vi "Window relative size to pixel size.vi"(8 "Border (px)":i16=4, 9 "Height (px)":i16=1920, 10 "Width (px)":i16=1920, 11 "Window Relative Size (%)":T2 {"Bottom (%)" format="%.2f"; "Top (%)" format="%.2f"; "Right (%)" format="%.2f"; "Left (%)" format="%.2f"}) -> (3 "16bit integer":T1)   [LabVIEW 2021, in "MultiStokePlot.lvlib" / "MultiPlotPanel.lvclass"]
uses:
  Classes/MultiPlotPanel/MultiPlotPanel.lvclass
  Window Position.ctl
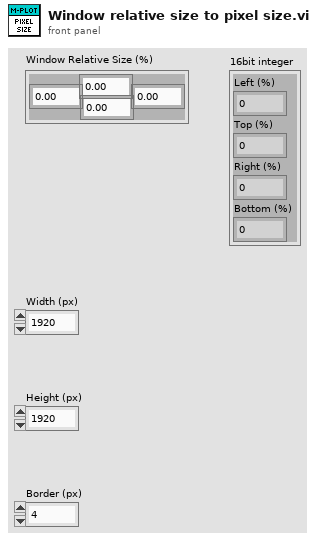
[diagram p1: front panel]
types:
  T1 = cluster{"Left (%)":i16, "Top (%)":i16, "Right (%)":i16, "Bottom (%)":i16}
  T2 = typedef "MultiStokePlot.lvlib/MultiPlotPanel.lvclass/Window Position.ctl" = cluster{"Left (%)":dbl, "Top (%)":dbl, "Right (%)":dbl, "Bottom (%)":dbl}
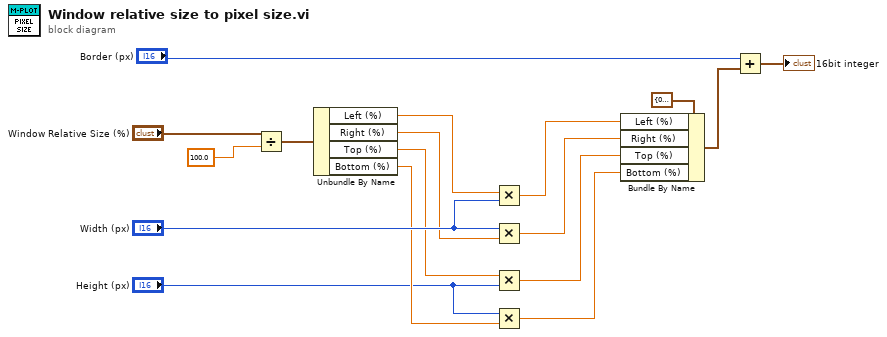
[diagram p0: block diagram]
diagram:
  n1 = Divide(x="Window Relative Size (%)", y=100.0 ("Right (%)")) -> (x/y=w15:T2)
  n2 = Unbundle By Name(w15) -> ("Left (%)"=w13:dbl, "Right (%)"=w7:dbl, "Top (%)"=w6:dbl, "Bottom (%)"=w10:dbl)
  n3 = Multiply(x=w13, y="Width (px)") -> (x*y=w4:dbl)
  n4 = Multiply(x="Width (px)", y=w7) -> (x*y=w11:dbl)
  n5 = Multiply(x=w6, y="Height (px)") -> (x*y=w5:dbl)
  n6 = Multiply(x="Height (px)", y=w10) -> (x*y=w8:dbl)
  n7 = Bundle By Name(cluster=T1 {"Left (%)"=0, "Top (%)"=0, "Right (%)"=43, "Bottom (%)"=13} ("16bit integer"), "Left (%)"=w4, "Right (%)"=w11, "Top (%)"=w5, "Bottom (%)"=w8) -> (w2:T1)
  n8 = Add(x="Border (px)", y=w2) -> (x+y=→"16bit integer":T1)
